vi "Port C LED AE.vi"() -> ()   [LabVIEW 2018]
uses:
  Port C AE LED type def.ctl
  <vilib>/Studica/Studica Toolkit/Background/DIO Channel.ctl
panel:
  out "DIO Info Out":T2
  out "error out":errorcluster
  in  "LED AE":T3
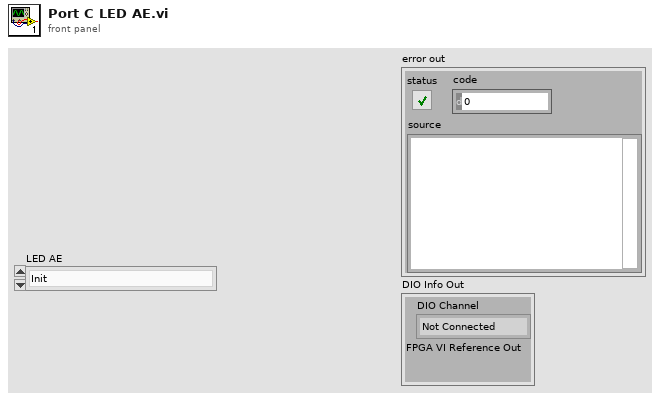
[diagram p1: front panel]
types:
  T1 = typedef "DIO Channel.ctl" = enum16{"Not Connected", "A/DIO1", "A/DIO2", "A/DIO3", "A/DIO4", "A/DIO5", "A/DIO6", "A/DIO7", "A/DIO13", "B/DIO1", "B/DIO2", "B/DIO3", "B/DIO4", "B/DIO5", "B/DIO6", "B/DIO7", "B/DIO13", "C/DIO0", "C/DIO1", "C/DIO2", "C/DIO3", "C/DIO4", "C/DIO5", "C/DIO6", "C/DIO7"}
  T2 = cluster{"DIO Channel":T1, "FPGA VI Reference Out":refnum<k20>}
  T3 = typedef "Port C AE LED type def.ctl" = enum16{"Init", "Green On", "Red On", "Both On", "Both Off", "Close"}
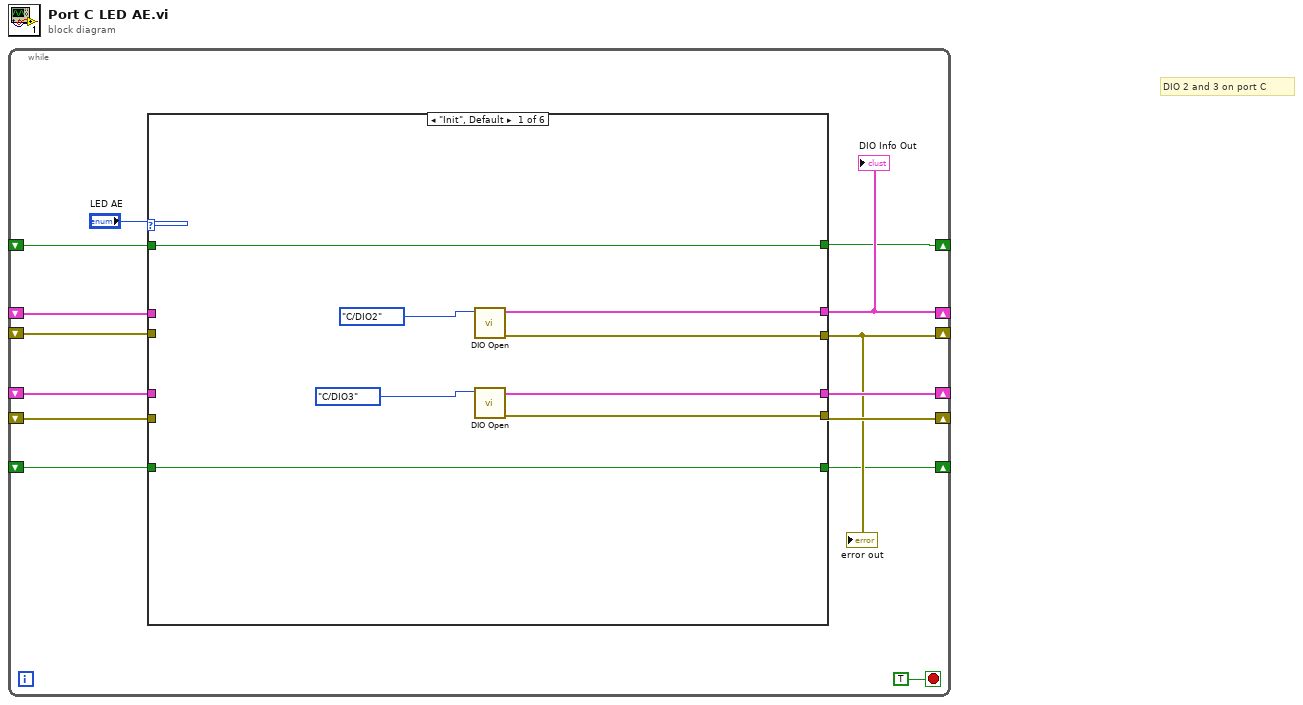
[diagram p0: block diagram]
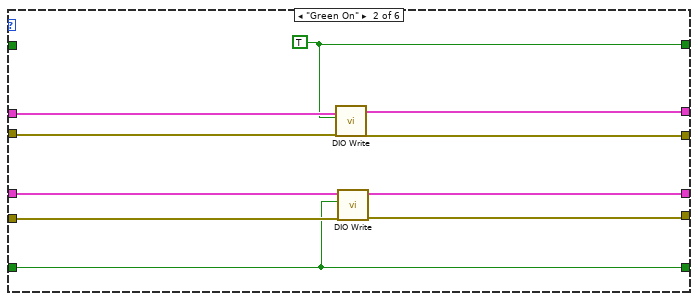
[diagram p2: hidden frame]
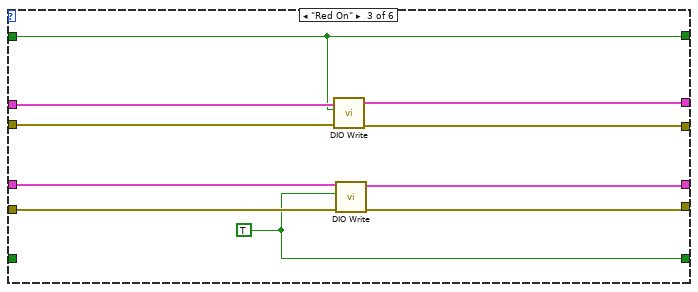
[diagram p3: hidden frame]
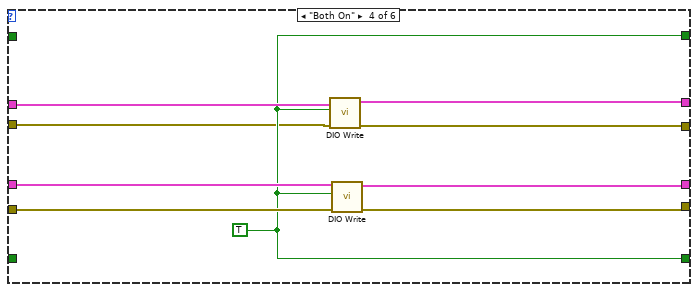
[diagram p4: hidden frame]
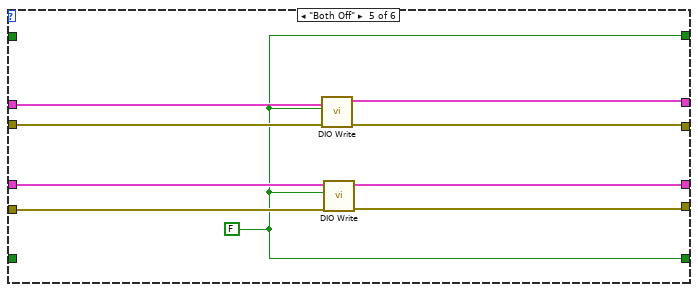
[diagram p5: hidden frame]
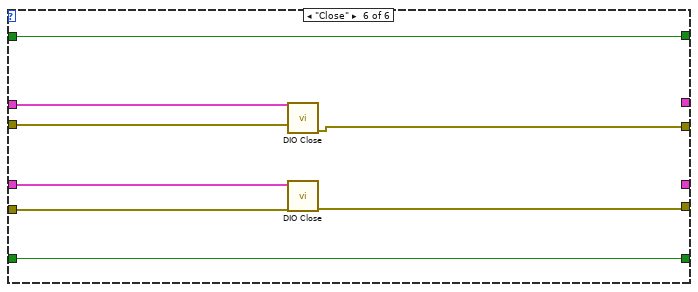
[diagram p6: hidden frame]
diagram:
  # "DIO 2 and 3 on port C"
  n1 = while {
    shift-right: [w12] -> _
    shift-left: _ -> [w9]
    shift-right: [w13] -> _
    shift-left: _ -> [w7]
    shift-right: [w11] -> _
    shift-left: _ -> [w6]
    shift-right: [w10] -> _
    shift-left: _ -> [w8]
    shift-right: [w5] -> _
    shift-left: _ -> [w4]
    shift-right: [w3] -> _
    shift-left: _ -> [w2]
    stop <- TRUE stop-if-true
    n2 = case shown="\"Init\", Default" "LED AE" {
      tunnel: [w20 w27 w37 w48 w58 _] -> w13
      tunnel: [w19 w30 w40 w50 w56 _] -> w12
      tunnel: [w18 w25 w35 w46 w57 w62] -> w11
      tunnel: [w17 w29 w39 w43 w55 w61] -> w10
      tunnel: w9 -> [_ w32 w42 w51 w54 w68]
      tunnel: w8 -> [_ w31 w41 w44 w53 w67]
      tunnel: w7 -> [_ w28 w38 w49 w60 w66]
      tunnel: w6 -> [_ w26 w36 w47 w59 w65]
      tunnel: [w16 w24 w34 w45 w52 w64] -> w5
      tunnel: w4 -> [w16 _ w34 _ _ w64]
      tunnel: [w15 w23 w33 w45 w52 w63] -> w3
      tunnel: w2 -> [w15 w23 _ _ _ w63]
      frame "Init", Default {
        n3 = call <vilib>:"DIO Open.vi"("DIO Channel"=DIO_Channel."C/DIO2") -> ("error out"=w17:errorcluster, "DIO Info Out"=w19:T2)  [unwired: 9 in]
        n4 = call <vilib>:"DIO Open.vi"("DIO Channel"=DIO_Channel."C/DIO3") -> ("error out"=w18:errorcluster, "DIO Info Out"=w20:T2)  [unwired: 9 in]
      }
      frame "Green On" {
        w24 = TRUE ("Input")
        n5 = call <vilib>:"DIO Write.vi"("error in (no error)"=w31, "Input"=w24, "DIO Info In"=w32) -> ("error out"=w29:errorcluster, "DIO Info Out"=w30:T2)  [unwired: 7 in]
        n6 = call <vilib>:"DIO Write.vi"("error in (no error)"=w26, "Input"=w23, "DIO Info In"=w28) -> ("error out"=w25:errorcluster, "DIO Info Out"=w27:T2)  [unwired: 7 in]
      }
      frame "Red On" {
        w33 = TRUE ("Input")
        n7 = call <vilib>:"DIO Write.vi"("error in (no error)"=w41, "Input"=w34, "DIO Info In"=w42) -> ("error out"=w39:errorcluster, "DIO Info Out"=w40:T2)  [unwired: 7 in]
        n8 = call <vilib>:"DIO Write.vi"("error in (no error)"=w36, "Input"=w33, "DIO Info In"=w38) -> ("error out"=w35:errorcluster, "DIO Info Out"=w37:T2)  [unwired: 7 in]
      }
      frame "Both On" {
        w45 = TRUE ("Input")
        n9 = call <vilib>:"DIO Write.vi"("error in (no error)"=w44, "Input"=w45, "DIO Info In"=w51) -> ("error out"=w43:errorcluster, "DIO Info Out"=w50:T2)  [unwired: 7 in]
        n10 = call <vilib>:"DIO Write.vi"("error in (no error)"=w47, "Input"=w45, "DIO Info In"=w49) -> ("error out"=w46:errorcluster, "DIO Info Out"=w48:T2)  [unwired: 7 in]
      }
      frame "Both Off" {
        w52 = FALSE ("Input")
        n11 = call <vilib>:"DIO Write.vi"("error in (no error)"=w53, "Input"=w52, "DIO Info In"=w54) -> ("error out"=w55:errorcluster, "DIO Info Out"=w56:T2)  [unwired: 7 in]
        n12 = call <vilib>:"DIO Write.vi"("error in (no error)"=w59, "Input"=w52, "DIO Info In"=w60) -> ("error out"=w57:errorcluster, "DIO Info Out"=w58:T2)  [unwired: 7 in]
      }
      frame "Close" {
        n13 = call <vilib>:"DIO Close.vi"("error in (no error)"=w67, "DIO Info In"=w68) -> ("error out"=w61:errorcluster)  [unwired: 9 in]
        n14 = call <vilib>:"DIO Close.vi"("error in (no error)"=w65, "DIO Info In"=w66) -> ("error out"=w62:errorcluster)  [unwired: 9 in]
      }
    }
    "error out" <- w10
    "DIO Info Out" <- w12
  }
